vi "DecimalDegreesToMeters.vi"(2 "Longitude":ext, 3 "Latitude":ext) -> (0 "X":dbl, 1 "Y":dbl)   [LabVIEW 2010]
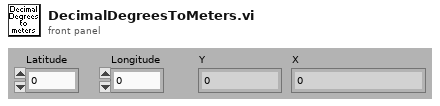
[diagram p1: front panel]
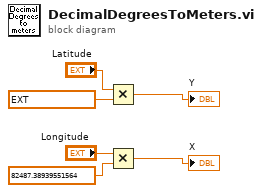
[diagram p0: block diagram]
diagram:
  n1 = Multiply(x="Latitude", y=ext 111078.68115990028 ("x")) -> (x*y=→"Y":ext)
  n2 = Multiply(x="Longitude", y=82487.38939551564 ("x")) -> (x*y=→"X":ext)
